vi "Offset From Base Buffer.vi"(8 "error in (no error)":errorcluster, 10 "base Buffer":refnum<class "Buffer.lvclass">, 11 "Buffer in":refnum<class "Buffer.lvclass">) -> (0 "error out":errorcluster, 3 "Buffer out":refnum<class "Buffer.lvclass">)   [LabVIEW 2017, in "DSF Core.lvlib" / "Buffer.lvclass"]
uses:
  Buffer.lvclass
  C:/Program Files (x86)/National Instruments/LabVIEW 2017/vi.lib/NI/Memory Manager/Classes/Pointer/Pointer.lvclass
  <vilib>/NI/Memory Manager/Classes/Pointer/Pointer.lvclass/Pointer.ctl
  Buffer.lvclass/Buffer.ctl
  <vilib>/NI/Memory Manager/Classes/Pointer/Set Size.vi
  <vilib>/NI/Memory Manager/Classes/Pointer/Set Address.vi
  <vilib>/NI/Memory Manager/Classes/Pointer/Check Null Pointer.vi
  <vilib>/NI/Memory Manager/Classes/Pointer/Set Internal.vi
  <vilib>/NI/Memory Manager/Classes/Pointer/Errors.vi
  <vilib>/NI/Memory Manager/Classes/Pointer/Null Pointer.vi
  <vilib>/NI/Memory Manager/Classes/Pointer/Create Error.vi
  <vilib>/NI/Memory Manager/VIs/New Error Cluster Constant.vi
  <vilib>/NI/Memory Manager/VIs/New Error Cluster Constant (512B).vi
  <vilib>/NI/Memory Manager/VIs/Error Cluster.Set Status.vi
  <vilib>/NI/Memory Manager/VIs/Error Cluster.Set Code.vi
  <vilib>/NI/Memory Manager/VIs/Error Cluster.Set VI Source.vi
  <vilib>/NI/Memory Manager/Constants/Constants.vi
  <vilib>/NI/Memory Manager/Constants/Library Name.vi
  <vilib>/NI/Memory Manager/Classes/Pointer/Pointer Error Info.vi
  <vilib>/NI/Memory Manager/VIs/Source.Write.String.vi
  <vilib>/NI/Memory Manager/Constants/Pointer Class Name.vi
  <vilib>/NI/Memory Manager/Classes/Pointer/Pointer.lvclass
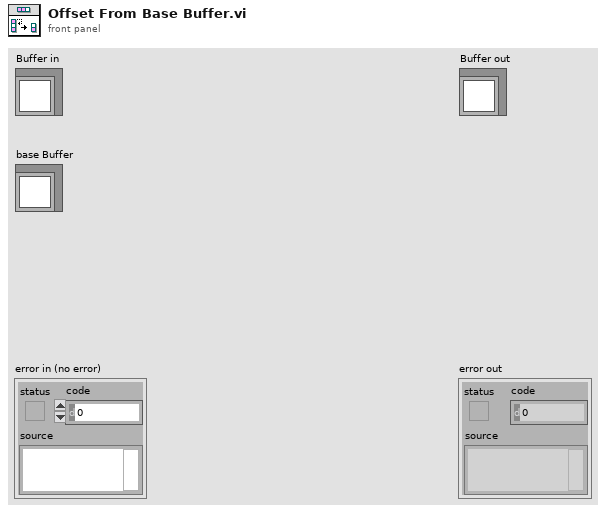
[diagram p1: front panel]
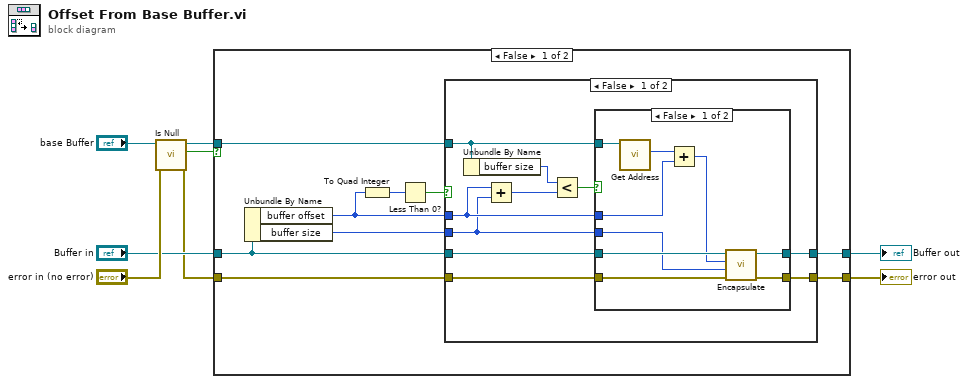
[diagram p0: block diagram]
diagram:
  n1 = call <vilib>:"Is Null.vi"("error in (no error)"="error in (no error)", "Pointer in"="base Buffer") -> ("error out"=w2:errorcluster, "null?"=w1:bool, "Pointer out"=w3:refnum<class "Buffer.lvclass">)  [unwired: 7 in]
  n2 = case shown="False" w1 {
    tunnel: [w17 w42] -> w8
    tunnel: [w16 w41] -> w7
    tunnel: w3 -> [w10 _]
    tunnel: "Buffer in" -> [w15 w42]
    tunnel: w2 -> [w9 w41]
    frame False {
      n3 = Unbundle By Name(w15) -> ("buffer offset"=w13:u64, "buffer size"=w14:u64)
      n4 = To Quad Integer(1:w13) -> (0:w12:i64)
      n5 = Less Than 0?(x=w12) -> (x < 0?=w11:bool)
      n6 = case shown="False" w11 {
        tunnel: [w27 w39] -> w17
        tunnel: [w26 w40] -> w16
        tunnel: w9 -> [w25 w40]
        tunnel: w15 -> [w24 w39]
        tunnel: w14 -> [w22 _]
        tunnel: w13 -> [w23 _]
        tunnel: w10 -> [w21 _]
        frame False {
          n7 = Unbundle By Name(w21) -> ("buffer size"=w20:u64)
          n8 = Add(x=w23, y=w22) -> (x+y=w19:u64)
          n9 = Less?(x=w20, y=w19) -> (x < y?=w18:bool)
          n10 = case shown="False" w18 {
            tunnel: [w36 w37] -> w27
            tunnel: [w35 w38] -> w26
            tunnel: w25 -> [w34 w38]
            tunnel: w24 -> [w33 w37]
            tunnel: w22 -> [w32 _]
            tunnel: w23 -> [w30 _]
            tunnel: w21 -> [w29 _]
            frame False {
              n11 = call <vilib>:"Get Address.vi"("Pointer in"=w29) -> ("address"=w28:u64)  [unwired: 9 in, 1 out]
              n12 = Add(x=w28, y=w30) -> (x+y=w31:u64)
              n13 = call <vilib>:"Encapsulate.vi"("error in (no error)"=w34, "size"=w32, "address"=w31, "Pointer in"=w33) -> ("error out"=w35:errorcluster, "Pointer out"=w36:refnum<class "Buffer.lvclass">)  [unwired: 6 in]
            }
            frame True {
              # "offset would be out of bounds of base buffer."
            }
          }
        }
        frame True {
          # "invalid offset"
        }
      }
    }
    frame True {
    }
  }
  "error out" <- w7
  "Buffer out" <- w8
